vi "ErrorMSG_message collector&reseter.vi"(0 "Warning List in":string[][](array[string]), 5 "Error List in":string[][](array[string]), 7 "Error reset":bool, 9 "dequeue timeout":bool, 11 "error &rester in":errorcluster, 12 "warning code header(2)":string="20") -> (2 "Warning Clear?":bool, 3 "Error Clear":bool, 4 "Warning List out":string[][](array[string]), 6 "Error List out":string[][](array[string]), 8 "Warning Expanded":bool, 10 "Error Expanded":bool)   [LabVIEW 2019]
doc: "This vi provides error/warning database write&reset,if any errors recieved,first it reconizes message which is \"error\" or \"warning\"by \"warning code header\",then write these messages into database and set a recieved time,you can use \"Error reset\" to reset any errors,for instance it'll clear all errors and write them into dababase including clear time without clear \"warnings\".the same you can clear warnings by set error state flag \"false\",gives the specific warning you want to clear by \"specific error code\" is given."
panel:
  in  "Error Code Length":i32=5
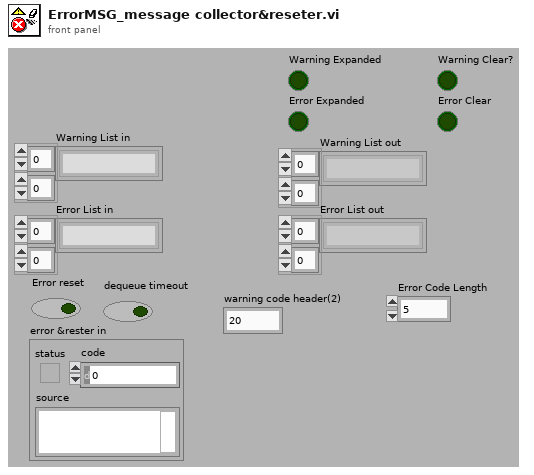
[diagram p1: front panel]
types:
  T1 = enum16{"idle", "error occurs", "warning occurs", "error cleared", "warning cleared", "run"}
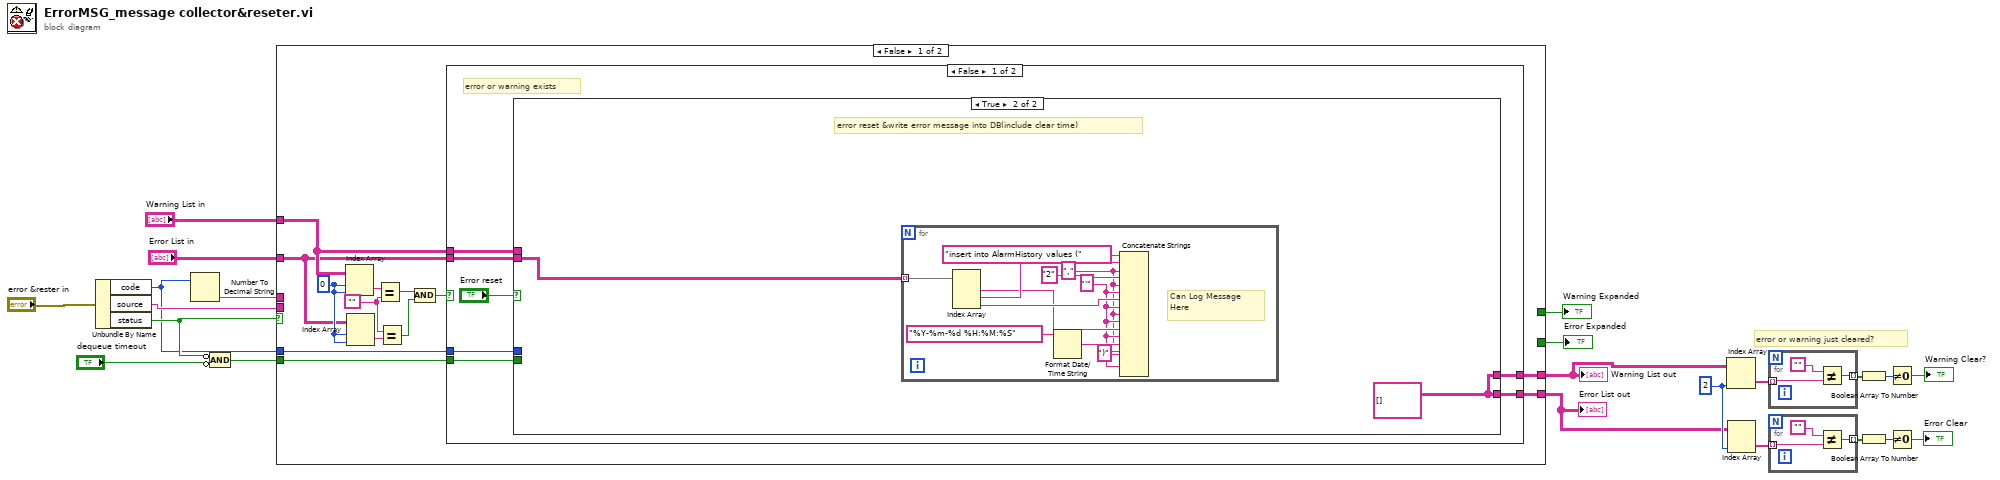
[diagram p0: block diagram]
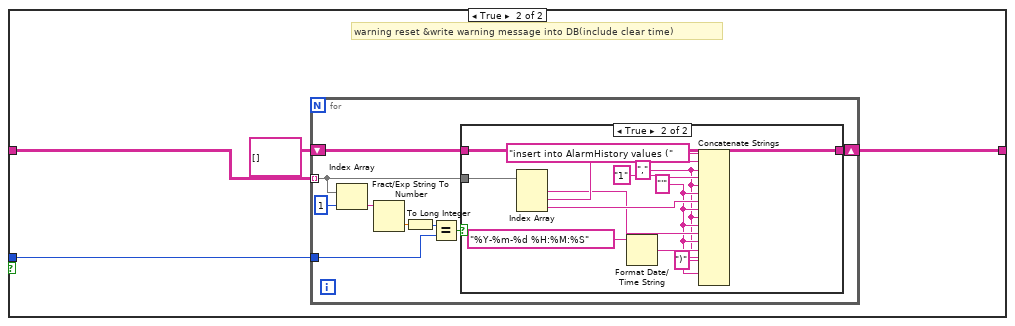
[diagram p3: hidden frame]
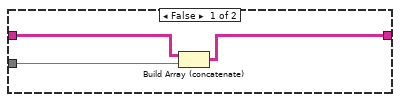
[diagram p4: hidden frame]
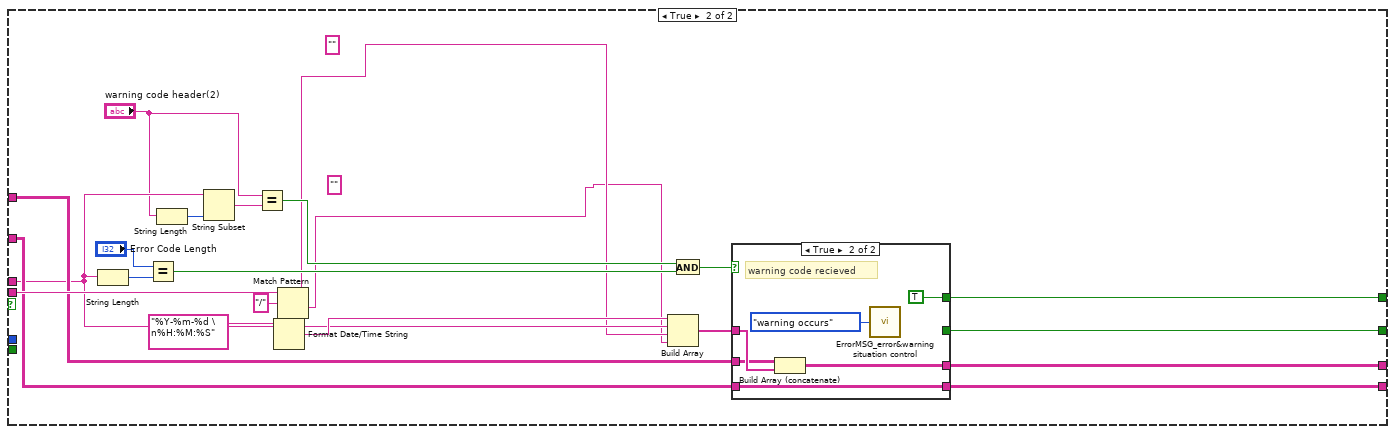
[diagram p6: hidden frame]
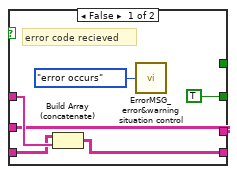
[diagram p7: hidden frame]
diagram:
  w7 = 2 ("disabled index (col)")
  # "error or warning just cleared?"
  n1 = Unbundle By Name("error &rester in") -> ("code"=w15:i32, "source"=w19:string, "status"=w17:bool)
  n2 = Number To Decimal String(number=w15) -> (decimal integer string=w14:string)  [unwired: 1 in]
  n3 = Compound Arithmetic op=AND(invert w17, invert "dequeue timeout") -> (w18:bool)
  n4 = case shown="False" w17 {
    tunnel: "Error List in" -> [w25 w105]
    tunnel: "Warning List in" -> [w29 w107]
    tunnel: w18 -> [w28 _]
    tunnel: w14 -> [_ w103]
    tunnel: w19 -> [_ w109]
    tunnel: [w26 w106] -> w4
    tunnel: [w24 w104] -> w3
    tunnel: w15 -> [w23 _]
    tunnel: [_ w95] -> w13
    tunnel: [_ w94] -> w12
    frame False {
      w30 = 0 ("index (row)")
      w33 = ""
      n5 = Index Array(array=w29, index (row)=w30, index (col)=w30) -> (element=w35:string)
      n6 = Index Array(array=w25, index (row)=w30, index (col)=w30) -> (element=w34:string)
      n7 = Equal?(x=w35, y=w33) -> (x = y?=w32:bool)
      n8 = Equal?(x=w33, y=w34) -> (x = y?=w31:bool)
      n9 = And(x=w32, y=w31) -> (x .and. y?=w27:bool)
      n10 = case shown="False" w27 {
        tunnel: w29 -> [w42 w91]
        tunnel: w28 -> [w41 _]
        tunnel: [w39 w91] -> w26
        tunnel: w25 -> [w37 w90]
        tunnel: [w38 w90] -> w24
        tunnel: w23 -> [w36 _]
        frame False {
          # "error or warning exists"
          n11 = case shown="True" "Error reset" {
            tunnel: w42 -> [w47 _]
            tunnel: w41 -> [w46 _]
            tunnel: [w45 w77] -> w39
            tunnel: [w43 w77] -> w38
            tunnel: w37 -> [w43 w78]
            tunnel: w36 -> [w44 _]
            frame False {
              n12 = case shown="False" w46 {
                tunnel: w47 -> [w48 w50]
                tunnel: [w48 w52] -> w45
                tunnel: w44 -> [_ w51]
                frame False {
                }
                frame True {
                  # "warning reset &write warning message into DB(include clear time)"
                  n13 = for {
                    tunnel: w50 -> [w57] mode=indexing
                    tunnel: w51 -> [w55]
                    shift-right: [w54] -> w52
                    shift-left: string[][] [] -> [w53]
                    n14 = Index Array(array=w57, index=1) -> (element=w56:string)
                    n15 = Fract/Exp String To Number(string=w56) -> (number=w60:dbl)  [unwired: 3 in, 1 out]
                    n16 = To Long Integer(number=w60) -> (32bit integer=w59:i32)
                    n17 = Equal?(x=w59, y=w55) -> (x = y?=w58:bool)
                    n18 = case shown="True" w58 {
                      tunnel: w57 -> [w64 w75]
                      tunnel: w53 -> [w63 w65]
                      tunnel: [w62 w65] -> w54
                      frame False {
                        n19 = Build Array (concatenate)(w63, w64) -> (w62:string[][])
                      }
                      frame True {
                        w70 = "'" ("string")
                        w66 = "," ("string")
                        n20 = Index Array(array=w75) -> (element #1=w72:string, element #2=w74:string, element #3=w73:string)  [unwired: 3 in]
                        n21 = Format Date/Time String(time format string (%c)="%Y-%m-%d %H:%M:%S") -> (date/time string=w71:string)  [unwired: 2 out]
                        n22 = Concatenate Strings("insert into AlarmHistory values (" ("string"), w74, w66, "1" ("string"), w66, w70, w73, w70, w66, w70, w72, w70, w66, w70, w71, w70, ")" ("string")) -> ()  [unwired: 1 out]
                      }
                    }
                  }
                }
              }
            }
            frame True {
              w77 = string[][] [] ("Item Names")
              # "error reset &write error message into DB(include clear time)"
              n23 = for {
                tunnel: w78 -> [w79] mode=indexing
                w84 = "'" ("string")
                w80 = "," ("string")
                # "Can Log Message\nHere"
                n24 = Index Array(array=w79) -> (element #1=w86:string, element #2=w88:string, element #3=w87:string)  [unwired: 3 in]
                n25 = Format Date/Time String(time format string (%c)="%Y-%m-%d %H:%M:%S") -> (date/time string=w85:string)  [unwired: 2 out]
                n26 = Concatenate Strings("insert into AlarmHistory values (" ("string"), w88, w80, "2" ("string"), w80, w84, w87, w84, w80, w84, w86, w84, w80, w84, w85, w84, ")" ("string")) -> ()  [unwired: 1 out]
              }
            }
          }
        }
        frame True {
          # "no errors or warnings"
        }
      }
    }
    frame True {
      (unwired) ""
      (unwired) ""
      n27 = String Length(string=w103) -> (length=w102:i32)
      n28 = Equal?(x="Error Code Length", y=w102) -> (x = y?=w97:bool)
      n29 = String Length(string="warning code header(2)") -> (length=w99:i32)
      n30 = String Subset(string=w103, length (rest)=w99) -> (substring=w113:string)  [unwired: 1 in]
      n31 = Equal?(x="warning code header(2)", y=w113) -> (x = y?=w98:bool)
      n32 = Format Date/Time String(time format string (%c)="%Y-%m-%d \n%H:%M:%S") -> (date/time string=w112:string)  [unwired: 2 out]
      n33 = Match Pattern(string=w109, regular expression="/") -> (before substring=w93:string, after substring=w92:string)  [unwired: 1 in, 2 out]
      n34 = Build Array(w112, w103, w93, w92) -> (w108:string[])
      n35 = And(x=w98, y=w97) -> (x .and. y?=w96:bool)
      n36 = case shown="True" w96 {
        tunnel: w108 -> [w119 w125]
        tunnel: w107 -> [w116 w124]
        tunnel: [w116 w123] -> w106
        tunnel: w105 -> [w118 w122]
        tunnel: [w117 w122] -> w104
        tunnel: [_ TRUE ("Warning Expanded")] -> w95
        tunnel: [TRUE ("Warning Expanded") _] -> w94
        frame False {
          # "error code recieved"
          n37 = Build Array (concatenate)(w118, w119) -> (w117:string[][])
          n38 = call "ErrorMSG_error&warning situation control.vi"("error&warning control"=T1."error occurs") -> ()  [unwired: 2 in]
        }
        frame True {
          # "warning code recieved"
          n39 = Build Array (concatenate)(w124, w125) -> (w123:string[][])
          n40 = call "ErrorMSG_error&warning situation control.vi"("error&warning control"=T1."warning occurs") -> ()  [unwired: 2 in]
        }
      }
    }
  }
  "Warning List out" <- w4
  "Error List out" <- w3
  "Error Expanded" <- w12
  "Warning Expanded" <- w13
  n41 = Index Array(array=w4, index (col)=w7) -> (element=w11:string[])  [unwired: 1 in]
  n42 = Index Array(array=w3, index (col)=w7) -> (element=w10:string[])  [unwired: 1 in]
  n43 = for {
    tunnel: w11 -> [w127] mode=indexing
    tunnel: [w126] -> w5 mode=indexing
    n44 = Not Equal?(x="", y=w127) -> (x != y?=w126:bool)
  }
  n45 = for {
    tunnel: w10 -> [w130] mode=indexing
    tunnel: [w129] -> w9 mode=indexing
    n46 = Not Equal?(x="", y=w130) -> (x != y?=w129:bool)
  }
  n47 = Boolean Array To Number(Boolean array=w5) -> (number=w6:u32)
  n48 = Boolean Array To Number(Boolean array=w9) -> (number=w8:u32)
  n49 = Not Equal To 0?(x=w6) -> (x != 0?=→"Warning Clear?":bool)
  n50 = Not Equal To 0?(x=w8) -> (x != 0?=→"Error Clear":bool)
